vi "Read Pot.vi"(7 "Output Type (Analog)":enum16{"Analog", "Digital"}(ring), 8 "error in (no error)":errorcluster, 10 "Axis In":T1=1 items=["Axis 1"=1, "Axis 2"=2, "Axis 3"=3, "Axis 4"=4, "Axis 5"=5, "Axis 6"=6, "Axis 7"=7, "Axis 8"=8], 11 "Board ID":T3=1 min=1 max=32 step=1) -> (0 "error out":errorcluster, 2 "Axis Out":T1=1 items=["Axis 1"=1, "Axis 2"=2, "Axis 3"=3, "Axis 4"=4, "Axis 5"=5, "Axis 6"=6, "Axis 7"=7, "Axis 8"=8], 3 "Bd ID Out":T2, 5 "Pot Voltage":dbl)   [LabVIEW 2010]
doc: "Reads the voltage value on the analog input channel corresponding to a given axis. \n\nOutput type:\nAnalog (default): Returns the ADC value converted to a floating point value between 0 and 5 corresponding to the potentiometer voltage\nDigital: Returns the ADC value of the potentiometer voltage\n\nNotes:\nADC value is retrieved from controller board by the \"Read ADC.vi\" included in the FlexMotion software library. This VI is effectively a wrapper to that function that allows the user to retrieve a value on an analog channel corresponding to a given axis number i.e. channel 1 for axis 1 with the additional nicety of a voltage conversion. In effect, this allows the developer to program like an ADC channel is tied to a certain axis although the FlexMotion software does not explicitly allow for this when the primary feedback type is not configured as analog.\n\nProper analog voltage conversion is dependent on the analog input channel ADC range being configured for 0-5V.\n\nWritten for the NI PCI-7350 series. Uses an estimated bias error that must be calibrated for a given controller."
uses:
  <vilib>/Motion/FlexMotion/CustomControls/CustomControls.llb/Axis To Control.flx
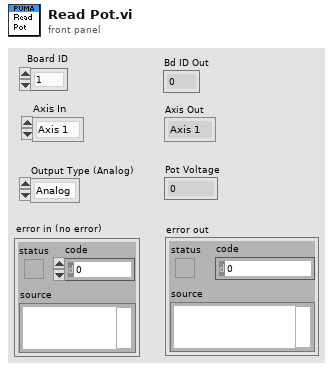
[diagram p1: front panel]
types:
  T1 = typedef "Axis To Control.flx" = u16
  T2 = typedef "Bd Id Out" = u8
  T3 = typedef "Board Id" = u8
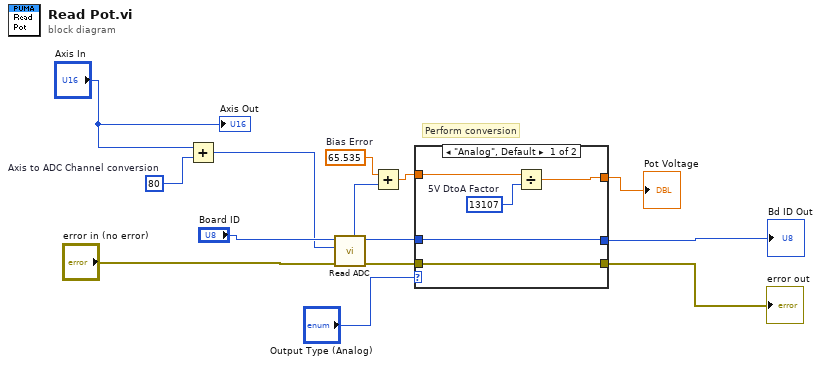
[diagram p0: block diagram]
diagram:
  w1 = 65.535  # Bias Error
  w6 = i16 80  # Axis to ADC Channel conversion
  # "Perform conversion"
  n1 = Add(x="Axis In", y=w6) -> (x+y=w4:T1)
  n2 = call <vilib>:"Read ADC.vi"("error in (no error)"="error in (no error)", "ADC"=w4, "Board ID"="Board ID") -> ("error out"=w10:errorcluster, "Bd ID Out"=w11:T2, "Analog Value"=w2:i32)  [unwired: 3 in, 1 out]
  n3 = Add(x=w1, y=w2) -> (x+y=w3:dbl)
  n4 = case shown="\"Analog\", Default" "Output Type (Analog)" {
    tunnel: w3 -> [w18 w20]
    tunnel: [w17 w20] -> w14
    tunnel: [w16 w22] -> w9
    tunnel: w11 -> [w16 w22]
    tunnel: [w15 w21] -> w8
    tunnel: w10 -> [w15 w21]
    frame "Analog", Default {
      w19 = 13107  # 5V DtoA Factor
      n5 = Divide(x=w18, y=w19) -> (x/y=w17:dbl)
    }
    frame "Digital" {
    }
  }
  "Pot Voltage" <- w14
  "Bd ID Out" <- w9
  "error out" <- w8
  "Axis Out" <- "Axis In"
